vi "notifyObserver.vi"(8 "error in (no error)":errorcluster, 11 "Subject.lvclass":refnum<class "Subject.lvclass">) -> (0 "error out":errorcluster, 3 "Subject.lvclass 2":refnum<class "Subject.lvclass">)   [LabVIEW 2020, in "Subject.lvclass"]
uses:
  Subject.lvclass
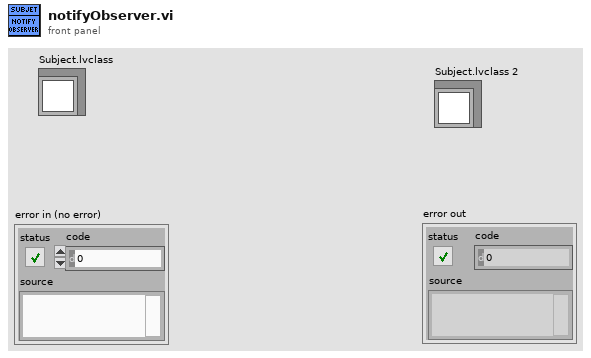
[diagram p1: front panel]
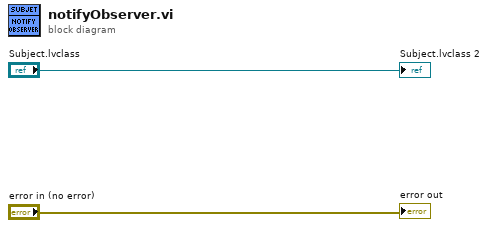
[diagram p0: block diagram]
diagram:
  "error out" <- "error in (no error)"
  "Subject.lvclass 2" <- "Subject.lvclass"
